vi "sensor_parameter_strict_type_to_strings.vi"(8 "error in (no error)":errorcluster, 10 "Sensor parameters":T1) -> (0 "error out":errorcluster, 2 "Sensor parameters (strings)":T2)   [LabVIEW 2018]
uses:
  sensor_parameters_strings.ctl
  sensor_parameters.ctl
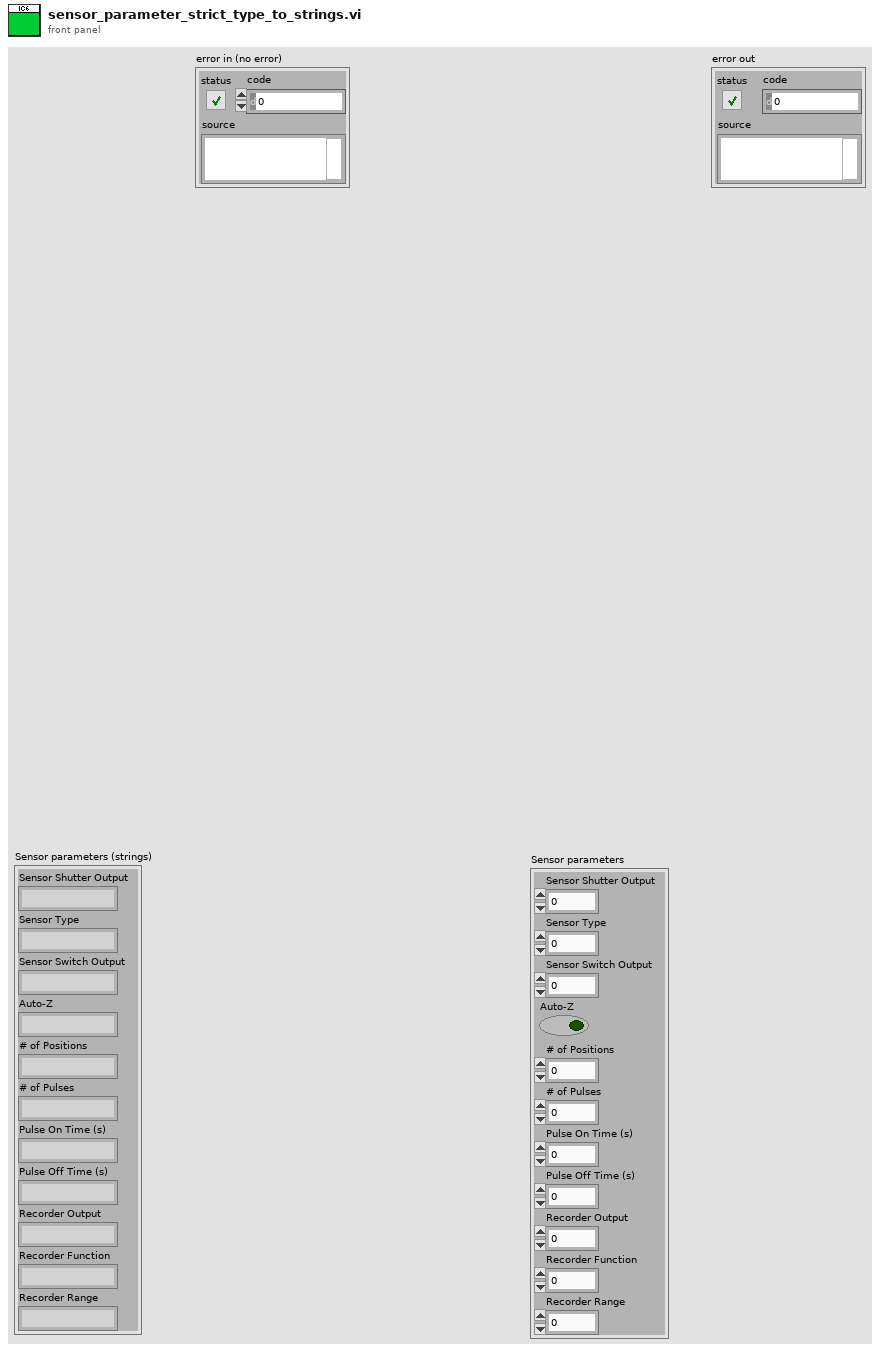
[diagram p1: front panel]
types:
  T1 = typedef "sensor_parameters.ctl" = cluster{"Sensor Shutter Output":u8, "Sensor Type":u8, "Sensor Switch Output":u8, "Auto-Z":bool, "# of Positions":u8, "# of Pulses":u8, "Pulse On Time (s)":sgl, "Pulse Off Time (s)":sgl, "Recorder Output":u8, "Recorder Function":u8, "Recorder Range":u32}
  T2 = typedef "sensor_parameters_strings.ctl" = cluster{"Sensor Shutter Output":string, "Sensor Type":string, "Sensor Switch Output":string, "Auto-Z":string, "# of Positions":string, "# of Pulses":string, "Pulse On Time (s)":string, "Pulse Off Time (s)":string, "Recorder Output":string, "Recorder Function":string, "Recorder Range":string}
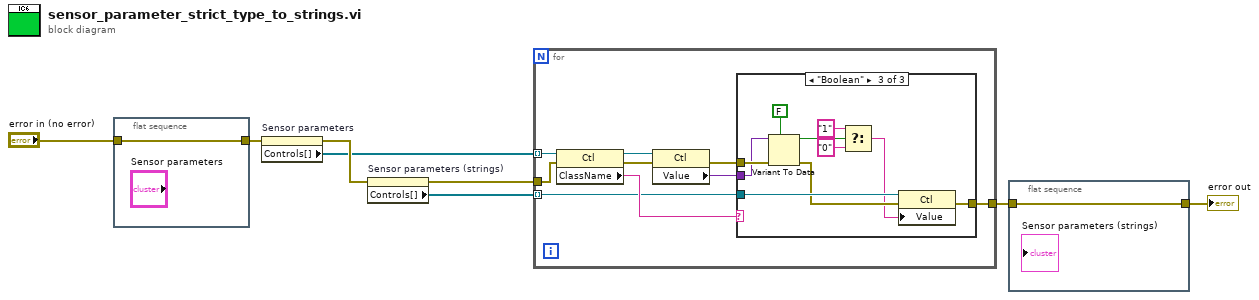
[diagram p0: block diagram]
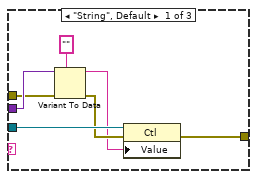
[diagram p2: hidden frame]
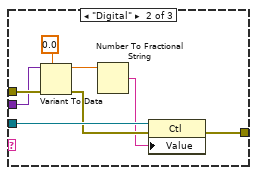
[diagram p3: hidden frame]
diagram:
  n1 = flat-sequence {
    tunnel: "error in (no error)" -> [w9]
    tunnel: [w9] -> w3
    frame #0 {
    }
  }
  n2 = property on="Sensor parameters" class="Clust (strict)"(error in=w3) -> (error out=w2:errorcluster, "Controls[]"=w1:refnum<vi>[])  [unwired: 1 in, 1 out]
  n3 = property on="Sensor parameters (strings)" class="Clust (strict)"(error in=w2) -> (error out=w4:errorcluster, "Controls[]"=w5:refnum<vi>[])  [unwired: 1 in, 1 out]
  n4 = for {
    tunnel: w1 -> [w12] mode=indexing
    tunnel: w5 -> [w10] mode=indexing
    tunnel: w4 -> [w18]
    tunnel: [w16] -> w7
    n5 = property class="Ctl"(reference=w12, error in=w18) -> (reference out=w11:refnum<vi>, error out=w17:errorcluster, "ClassName"=w13:string)
    n6 = property class="Ctl"(reference=w11, error in=w17) -> (error out=w15:errorcluster, "Value"=w14:variant)  [unwired: 1 out]
    n7 = case shown="\"Boolean\"" w13 {
      tunnel: w10 -> [w24 w33 w43]
      tunnel: [w25 w32 w42] -> w16
      tunnel: w15 -> [w22 w30 w41]
      tunnel: w14 -> [w23 w29 w40]
      frame "String", Default {
        n8 = Variant To Data(error in=w22, type="", Variant=w23) -> (data=w19:string, error out=w20:errorcluster)
        n9 = property class="Ctl"(reference=w24, error in=w20, "Value"=w19) -> (error out=w25:errorcluster)  [unwired: 1 out]
      }
      frame "Digital" {
        n10 = Variant To Data(error in=w30, type=0.0, Variant=w29) -> (data=w27:dbl, error out=w28:errorcluster)
        n11 = Number To Fractional String(number=w27) -> (F-format string=w26:string)  [unwired: 3 in]
        n12 = property class="Ctl"(reference=w33, error in=w28, "Value"=w26) -> (error out=w32:errorcluster)  [unwired: 1 out]
      }
      frame "Boolean" {
        n13 = Variant To Data(error in=w41, type=FALSE, Variant=w40) -> (data=w37:bool, error out=w39:errorcluster)
        n14 = Select(t="1", s=w37, f="0") -> (s? t:f=w34:string)
        n15 = property class="Ctl"(reference=w43, error in=w39, "Value"=w34) -> (error out=w42:errorcluster)  [unwired: 1 out]
      }
    }
  }
  n16 = flat-sequence {
    tunnel: w7 -> [w44]
    tunnel: [w44] -> w6
    frame #0 {
    }
  }
  "error out" <- w6
